vi "SPI read.vi"(8 "error in":errorcluster, 10 "SPI Address":u16, 11 "FPGA SPI config ref":T1) -> (0 "error out":errorcluster, 2 "IO Module\\SPI Read Data":u8, 3 "FPGA SPI config out":T1)   [LabVIEW 2013]
uses:
  FPGA_spi_config.ctl
  <vilib>/rvi/interface/common/niFpgaWaitOnOcc.vi
  <vilib>/Utility/error.llb/Error Cluster From Error Code.vi
  <vilib>/rvi/errors/niLvFpgaAdjustHostInterfaceError.vi
  <vilib>/rvi/interface/nirviReadWriteControl/nirviReadWriteControl.xnode
  NiFpgaLv.dll
  <vilib>/rvi/interface/Simulation/niFpgaSimulationCallBeginRW.vi
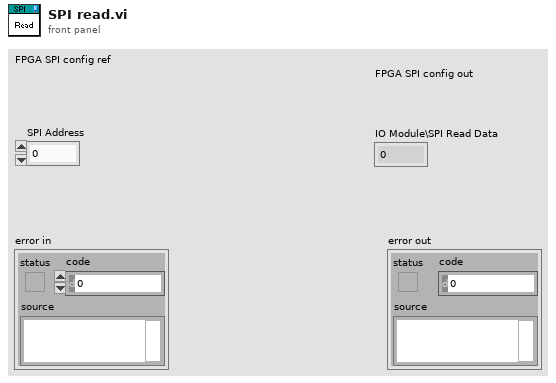
[diagram p1: front panel]
types:
  T1 = typedef "FPGA_spi_config.ctl" = refnum<k20>
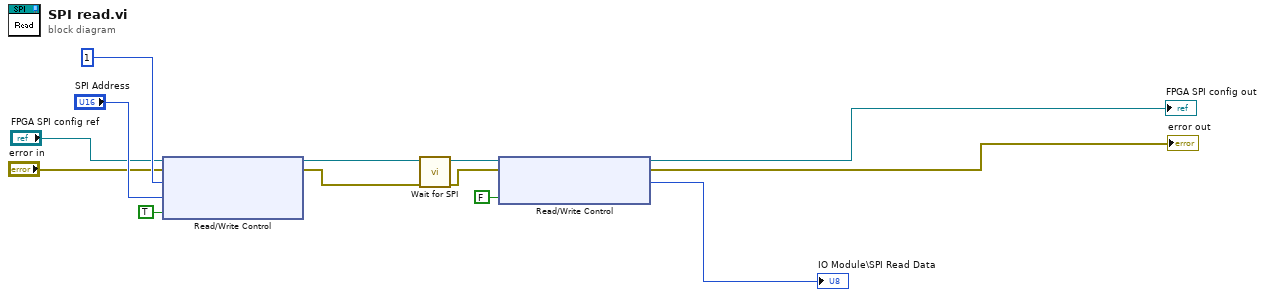
[diagram p0: block diagram]
diagram:
  n1 = xnode "Read/Write Control"("FPGA VI Reference In"="FPGA SPI config ref", "error in"="error in", "IO Module\\SPI Device"=u8 1 ("IO Module\\SPI Device"), "IO Module\\SPI Address"="SPI Address", "IO Module\\SPI Read"=TRUE ("IO Module\\SPI Read")) -> ("FPGA VI Reference Out"=w12:T1, "error out"=w11:errorcluster)
  n2 = call "Wait for SPI.vi"("error in"=w11, "FPGA SPI config ref"=w12) -> ("error out"=w9:errorcluster, "FPGA SPI config out"=w10:T1)  [unwired: 7 in, 1 out]
  n3 = xnode "Read/Write Control"("FPGA VI Reference In"=w10, "error in"=w9, "IO Module\\SPI Read"=FALSE ("IO Module\\SPI Read")) -> ("FPGA VI Reference Out"=→"FPGA SPI config out":T1, "error out"=→"error out":errorcluster, "IO Module\\SPI Read Data"=→"IO Module\\SPI Read Data":u8)
